vi "Log Actions.vi"(8 "error in":errorcluster, 10 "Clear Log":bool, 11 "Action":string="a") -> (0 "error out":errorcluster, 2 "Array":cluster{"Action":string, "Time":string}[](array[cluster]), 3 "Action Out":string="a")   [LabVIEW 2015]
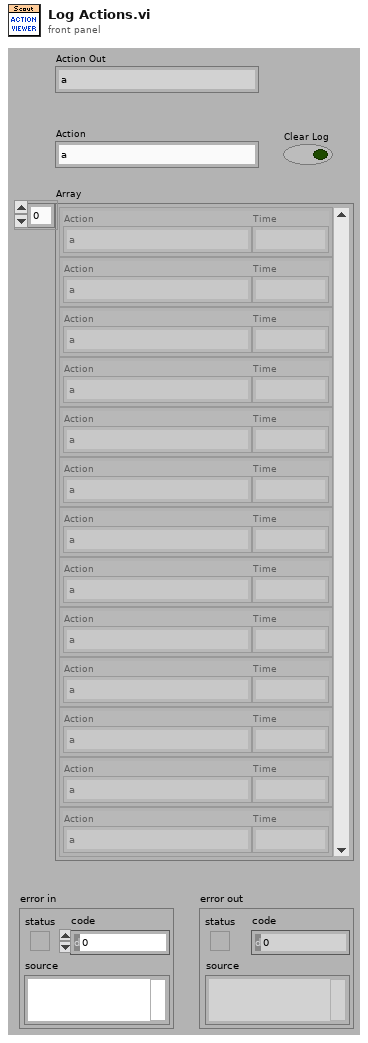
[diagram p1: front panel]
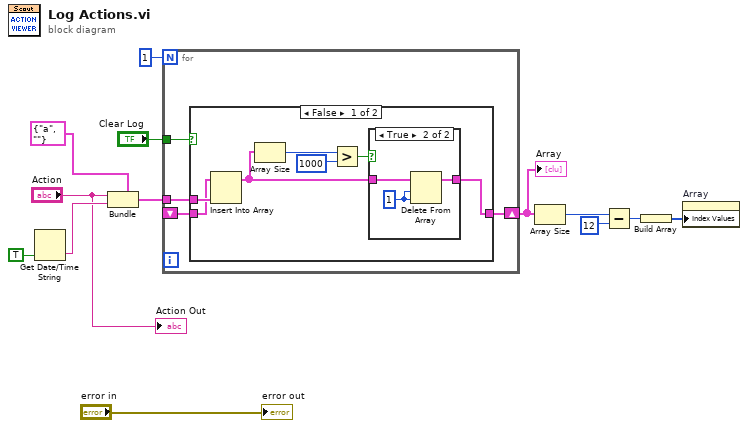
[diagram p0: block diagram]
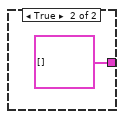
[diagram p3: hidden frame]
diagram:
  n1 = Get Date/Time String(want seconds? (F)=TRUE) -> (time string=w11:string)  [unwired: 2 in, 1 out]
  n2 = Bundle(cluster=cluster{"Action":string, "Time":string} {"Action"="a", "Time"=""} ("Cluster"), "Action"="Action", "Time"=w11) -> (w10:cluster{"Action":string, "Time":string})
  n3 = for {
    N: 1 -> [_]
    shift-right: [w15] -> w8
    shift-left: _ -> [w16]
    tunnel: w10 -> [w17]
    tunnel: "Clear Log" -> [w14]
    n4 = case shown="False" w14 {
      tunnel: w17 -> [w24 _]
      tunnel: w16 -> [w23 _]
      tunnel: [w22 cluster{"Action":string, "Time":string}[] []] -> w15
      frame False {
        n5 = Insert Into Array(array=w23, new element=w24) -> (w21:cluster{"Action":string, "Time":string}[])  [unwired: 1 in]
        n6 = Array Size(array=w21) -> (size(s)=w20:i32)
        n7 = Greater?(x=w20, y=1000) -> (0:w18:bool)
        n8 = case shown="True" w18 {
          tunnel: [w25 w28] -> w22
          tunnel: w21 -> [w25 w27]
          frame False {
          }
          frame True {
            w26 = 1 ("index")
            n9 = Delete From Array(array=w27, length=w26, index=w26) -> (array with subset deleted=w28:cluster{"Action":string, "Time":string}[])  [unwired: 1 out]
          }
        }
      }
      frame True {
      }
    }
  }
  "Array" <- w8
  n10 = Array Size(array=w8) -> (size(s)=w5:i32)
  n11 = Subtract(x=w5, y=12) -> (x-y=w6:i32)
  n12 = Build Array(w6) -> (w7:i32[])
  n13 = property on="Array" class="Arr (strict)"("Index Values"=w7) -> ()  [unwired: 2 in, 2 out]
  "error out" <- "error in"
  "Action Out" <- "Action"
